vi "Write Data_HoldingRegistors.vi"(6 "Index":i32, 8 "error in (no error)":errorcluster, 9 "register values":dbl[](array[numeric]), 11 "Device in":refnum<class "RS232_Device.lvclass">) -> (0 "error out":errorcluster, 3 "Device out":refnum<class "RS232_Device.lvclass">)   [LabVIEW 2023, in "RS232_Device.lvclass"]
uses:
  RS232_Device.lvclass
  D:/SamparkProdLine/subVIs/DAQ Device/Modbus_Device/DAQ_Device.lvclass
  RS232_Device.lvclass/RS232_Device.ctl
  <vilib>/Utility/error.llb/Trim Whitespace One-Sided.vi
panel:
  out "x = y?":bool
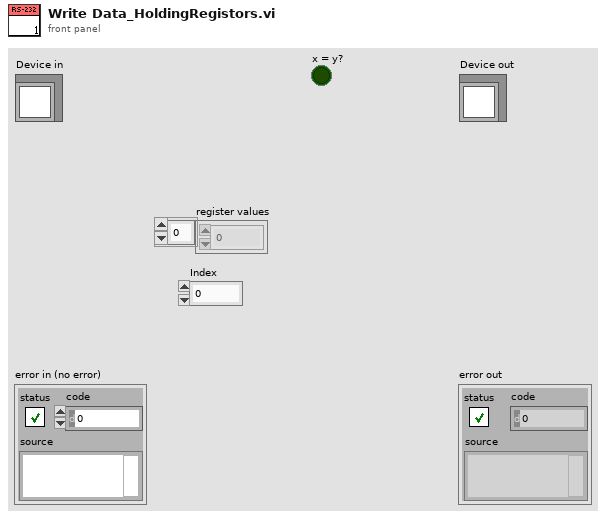
[diagram p1: front panel]
types:
  T1 = typedef "DAQ Device_IO ChannelsData.ctl" = cluster{"#DigitalInputs":u16, "StartAddress_DI":u16, "#DigitalOutputs":u16, "StartAddress_DO":u16, "#AnalogInputs":u16, "StartAddress_AI":u16, "#AnalogOutputs":u16, "StartAddress_AO":u16, "Coil_ReadData":bool[], "Coil_WriteData":bool[], "AI_Data":u16[], "AO_Data":u16[]}
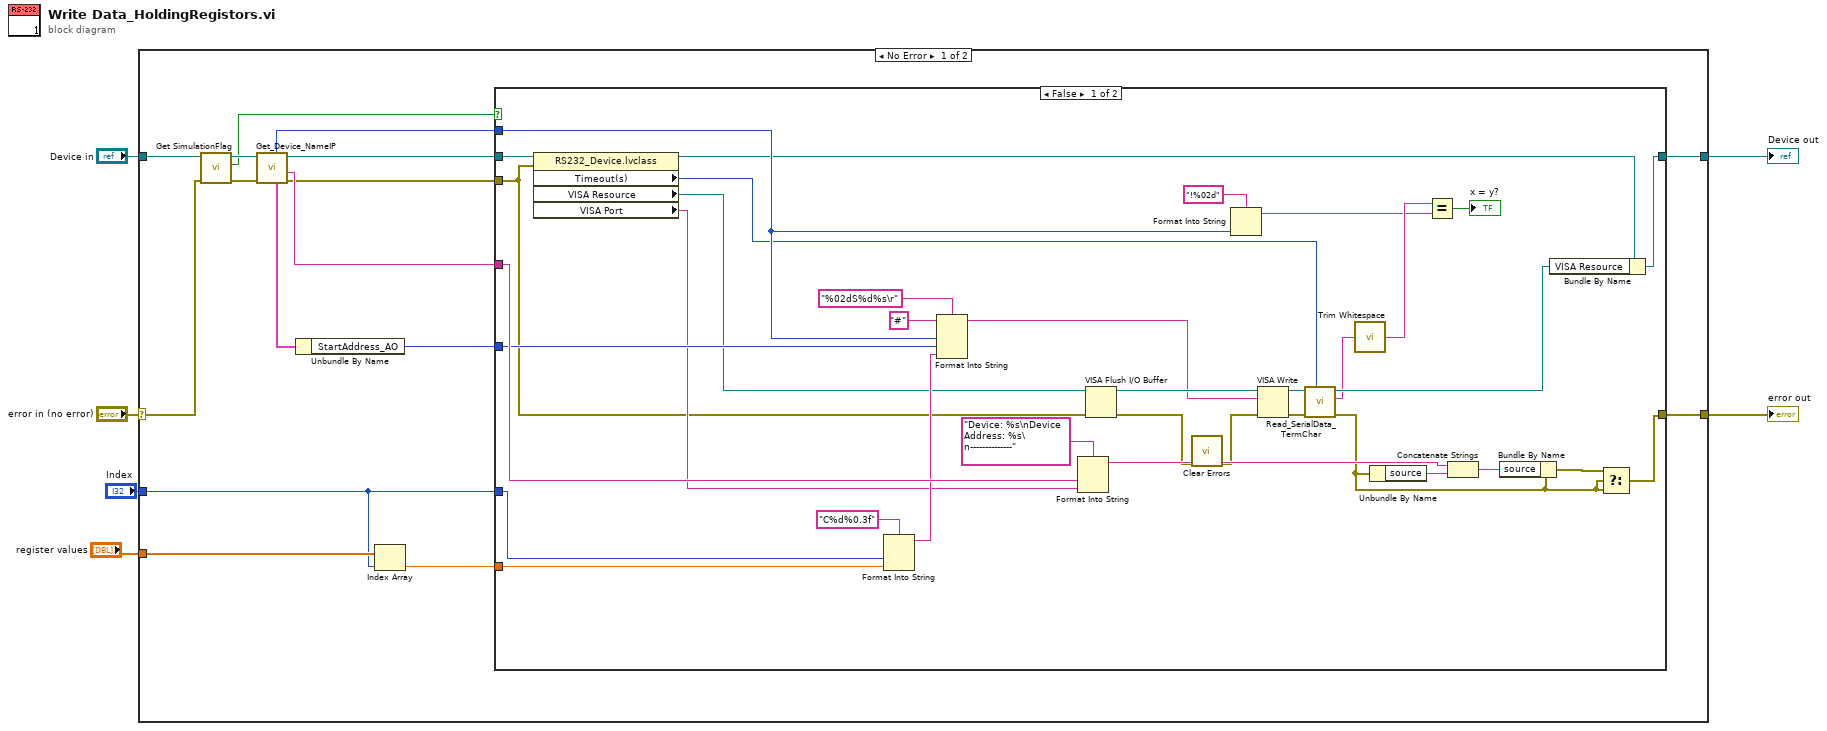
[diagram p0: block diagram]
diagram:
  n1 = case shown="No Error" "error in (no error)" {
    selector: "error in (no error)" -> [w7 w61]
    tunnel: [w21 w61] -> w3
    tunnel: [w22 w60] -> w5
    tunnel: "Device in" -> [w14 w60]
    tunnel: "register values" -> [w20 _]
    tunnel: "Index" -> [w18 _]
    frame No Error {
      n2 = call-dynamic "Get SimulationFlag.vi"("error in (no error)"=w7, "Device in"=w14) -> ("error out"=w17:errorcluster, "Simulation?"=w11:bool, "Device out"=w16:refnum<class "RS232_Device.lvclass">)  [unwired: 7 in]
      n3 = call-dynamic "Get_Device_NameIP.vi"("error in (no error)"=w17, "Device in"=w16) -> ("error out"=w8:errorcluster, "Device Name"=w12:string, "Device out"=w9:refnum<class "RS232_Device.lvclass">, "IO Channels"=w15:T1, "Unit ID"=w13:u8)  [unwired: 4 in, 1 out]
      n4 = Unbundle By Name(w15) -> ("StartAddress_AO"=w10:u16)
      n5 = Index Array(array=w20, index=w18) -> (element=w19:dbl)
      n6 = case shown="False" w11 {
        tunnel: [w23 w59] -> w22
        tunnel: [w57 w58] -> w21
        tunnel: w12 -> [w56 _]
        tunnel: w13 -> [w34 _]
        tunnel: w10 -> [w41 _]
        tunnel: w19 -> [w37 _]
        tunnel: w18 -> [w36 _]
        tunnel: w9 -> [w29 w59]
        tunnel: w8 -> [w24 w58]
        frame False {
          n7 = property class="RS232_Device.lvclass"(reference=w29, error in=w24) -> (reference out=w28:refnum<class "RS232_Device.lvclass">, "Timeout(s)"=w27:i32, "VISA Resource"=w26:refnum<visa-resource-name>, "VISA Port"=w25:string)  [unwired: 1 out]
          n8 = Format Into String(format string="C%d%0.3f", w36, w37) -> (resulting string=w38:string)  [unwired: 2 in, 1 out]
          n9 = Format Into String(format string="%02dS%d%s\r", initial string="#", w34, w41, w38) -> (resulting string=w40:string)  [unwired: 1 in, 1 out]
          n10 = Format Into String(format string="Device: %s\nDevice Address: %s\n--------------", w56, w25) -> (resulting string=w52:string)  [unwired: 2 in, 1 out]
          n11 = VISA Flush I/O Buffer(VISA resource name=w26, error in (no error)=w24) -> (VISA resource name out=w50:refnum<visa-resource-name>, error out=w49:errorcluster)  [unwired: 1 in]
          n12 = call <vilib>:"Clear Errors.vi"("error in (no error)"=w49) -> ("error out"=w48:errorcluster)  [unwired: 5 in, 1 out]
          n13 = Format Into String(format string="!%02d" ("regular expression"), w34) -> (resulting string=w31:string)  [unwired: 2 in, 1 out]
          n14 = VISA Write(VISA resource name=w50, write buffer=w40, error in (no error)=w48) -> (VISA resource name out=w47:refnum<visa-resource-name>, error out=w46:errorcluster)  [unwired: 1 out]
          n15 = call "Read_SerialData_TermChar.vi"("timeout (50ms)"=w27, "error in (no error)"=w46, "VISA Refnum in"=w47) -> ("error out"=w45:errorcluster, "StringData"=w33:string, "VISA Refnum out"=w44:refnum<visa-resource-name>)  [unwired: 6 in]
          n16 = call <vilib>:"Trim Whitespace.vi"("string"=w33) -> ("trimmed string"=w32:string)  [unwired: 1 in]
          n17 = Unbundle By Name(w45) -> ("source"=w54:string)
          n18 = Equal?(x=w32, y=w31) -> (x = y?=→"x = y?":bool)
          n19 = Concatenate Strings(w52, w54) -> (w51:string)
          n20 = Bundle By Name(cluster=w45, "source"=w51) -> (w55:errorcluster)
          n21 = Bundle By Name(cluster=w28, "VISA Resource"=w44) -> (w23:refnum<class "RS232_Device.lvclass">)
          n22 = Select(t=w55, s=w45, f=w45) -> (s? t:f=w57:errorcluster)
        }
        frame True {
        }
      }
    }
    frame Error {
    }
  }
  "error out" <- w3
  "Device out" <- w5
